vi "Configure Horizontal.vi"(8 "error in":errorcluster, 11 "DS1054 Base CFG in":refnum<class "DS1054 Base CFG.lvclass">) -> (0 "error out":errorcluster, 3 "DS1054 Base CFG out":refnum<class "DS1054 Base CFG.lvclass">)   [LabVIEW 2023, in "HAL.lvlib" / "RIGOL DS1054Z.lvlib" / "DS1054 Base CFG.lvclass"]
uses:
  DS1054 Base CFG.lvclass
  DS1054 Base CFG.lvclass/DS1054 Base CFG.ctl
  Configuration Base/Configuration Base.lvclass
  Scope VISA/Configuration/Scope VISA CFG.lvclass
  <instrlib>/RIGOL-DS1054Z-LabVIEW/RIGOL DS1054Z Driver.lvlib
  <vilib>/JDP Science/JSONtext/JSONtext.lvlib
  00f37b74-1b8e-44d6-87ce-f24b75bb551c.vi
  6a25d16a-339e-4ab2-87b2-bffc9528a97e.vi
  <vilib>/ErrorRing/Error Ring.xnode
  <vilib>/Utility/error.llb/Error Cluster From Error Code.vi
  d60901bd-e174-4fb7-b4eb-6ae63ce48c6a.vi
  D:/git/HAL/Scope VISA/Configuration/Scope VISA CFG.lvclass
  D:/git/HAL/Configuration Base/Configuration Base.lvclass
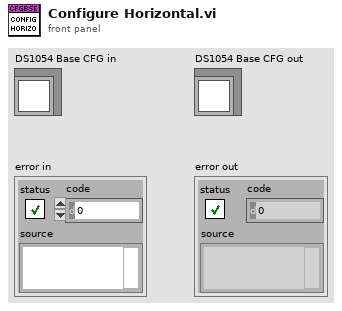
[diagram p1: front panel]
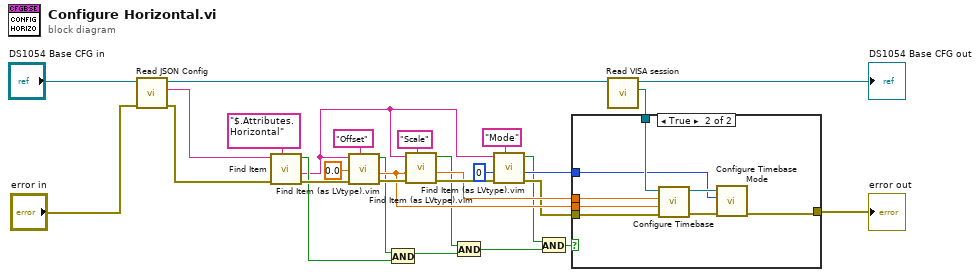
[diagram p0: block diagram]
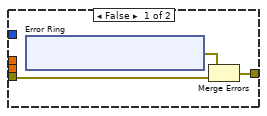
[diagram p2: hidden frame]
diagram:
  n1 = call "Read JSON Config.vi"("error in"="error in", "object in"="DS1054 Base CFG in") -> ("error out"=w22:errorcluster, "<JSON>Config"=w27:string, "object out"=w25:refnum<class "DS1054 Base CFG.lvclass">)  [unwired: 7 in]
  n2 = call <vilib>:"Find Item.vi"("$Path or Item Name"="$.Attributes.Horizontal", "error in (no error)"=w22, "JSON"=w27) -> ("error out"=w21:errorcluster, "<JSON>"=w1:string, "Found"=w13:bool)  [unwired: 5 in, 1 out]
  n3 = call "Find Item (as LVtype).vim"("$Path or Item Name"="Offset", "error in (no error)"=w21, "Data Type and Default Value"=0.0, "JSON"=w1) -> ("error out"=w19:errorcluster, "Data"=w14:dbl, "Found"=w12:bool)  [unwired: 4 in, 1 out]
  n4 = And(x=w12, y=w13) -> (x .and. y?=w10:bool)
  n5 = call "Find Item (as LVtype).vim"("$Path or Item Name"="Scale", "error in (no error)"=w19, "Data Type and Default Value"=w14, "JSON"=w1) -> ("error out"=w16:errorcluster, "Data"=w15:dbl, "Found"=w11:bool)  [unwired: 4 in, 1 out]
  n6 = And(x=w11, y=w10) -> (x .and. y?=w3:bool)
  n7 = call "Find Item (as LVtype).vim"("$Path or Item Name"="Mode", "error in (no error)"=w16, "Data Type and Default Value"=u16 0, "JSON"=w1) -> ("error out"=w8:errorcluster, "Data"=w5:u16, "Found"=w2:bool)  [unwired: 4 in, 1 out]
  n8 = And(x=w2, y=w3) -> (x .and. y?=w4:bool)
  n9 = call "Read VISA session.vi"("Scope VISA CFG in"=w25) -> ("VISA session"=w23:refnum<visa-resource-name>, "Scope VISA CFG out"=→"DS1054 Base CFG out":refnum<class "DS1054 Base CFG.lvclass">)  [unwired: 8 in, 1 out]
  n10 = case shown="True" w4 {
    tunnel: w23 -> [_ w45]
    tunnel: w8 -> [w31 w42]
    tunnel: w15 -> [_ w41]
    tunnel: w14 -> [_ w40]
    tunnel: [w30 w38] -> w9
    tunnel: w5 -> [_ w39]
    frame False {
      n11 = xnode "Error Ring"() -> ("error out"=w32:errorcluster)
      n12 = Merge Errors(w32, w31) -> (w30:errorcluster)
    }
    frame True {
      n13 = call <instrlib>:"Configure Timebase.vi"("error in (no error)"=w42, "Offset (0.0 s)"=w40, "Timebase (0.0005 s)"=w41, "VISA resource name"=w45) -> ("error out"=w43:errorcluster, "VISA resource name out"=w44:refnum<visa-resource-name>)  [unwired: 6 in]
      n14 = call <instrlib>:"Configure Timebase Mode.vi"("error in (no error)"=w43, "Timebase Mode (0: YT)"=w39, "VISA resource name"=w44) -> ("error out"=w38:errorcluster)  [unwired: 7 in, 1 out]
    }
  }
  "error out" <- w9
